vi "iIR.vi"(11 "PID gains":T1={"proportional gain (Kc)"=1.0, "integral time (Ti, min)"=0.01, "derivative time (Td, min)"=0.0} {"derivative time (Td, min)" format="%.4f"; "integral time (Ti, min)" format="%.3f"; "proportional gain (Kc)" format="%.3f"}) -> (2 "IR value":dbl[](array[numeric]), 9 "誤差":dbl)   [LabVIEW 2018]
uses:
  <vilib>/Platform/TimedLoop/XDataNode/timing_clust.ctl
  <vilib>/Platform/TimedLoop/XDataNode/nitl_modes.ctl
  <vilib>/Platform/TimedLoop/XDataNode/wakeup.ctl
  <vilib>/myRIO/Common/Instrument Driver Framework/myRIO v1.0/UART/vis/myRIO v1.0 Close UART.vi
  <vilib>/addons/control/pid/pid.llb/PID (DBL).vi
  <vilib>/myRIO/Common/Instrument Driver Framework/Utilities/vis/FPGA Ref Manager.vi
  <vilib>/myRIO/Common/Instrument Driver Framework/myRIO v1.0/myRIO v1.0 Reset FPGA.vi
  <vilib>/myRIO/Common/Instrument Driver Framework/myRIO v1.0/IRQ/vis/myRIO v1.0 IRQ Info FGV.vi
  <vilib>/myRIO/Common/Instrument Driver Framework/myRIO v1.0/IRQ/vis/myRIO v1.0 Timer IRQ Info FGV.vi
  <vilib>/myRIO/Common/Instrument Driver Framework/myRIO v1.0/IRQ/vis/myRIO v1.0 ISR Agent.vi
  <vilib>/platform/TimedLoop/XDataNode/XDataNode.xnode
  <vilib>/addons/control/pid/NI_PID_pid.lvlib
  <vilib>/Platform/TimedLoop/XDataNode/XDNodeRunTimeDep.lvlib
  <vilib>/myRIO/Instrument Drivers/Utilities/Utilities.lvlib
panel:
  in  "stop":bool
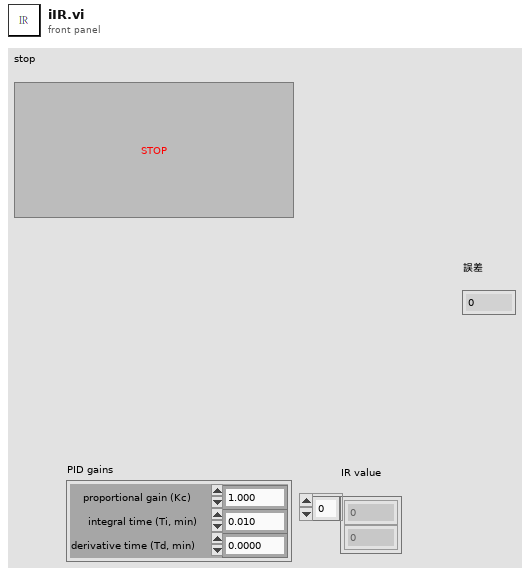
[diagram p1: front panel]
types:
  T1 = cluster{"proportional gain (Kc)":dbl, "integral time (Ti, min)":dbl, "derivative time (Td, min)":dbl}
  T2 = typedef "XDNodeRunTimeDep.lvlib/timing_clust.ctl" = cluster{"Expected End [f-1]":u64, "Actual End [f-1]":u64, "Finished Late? [f-1]":bool, "Expected End [i-1]":u64, "Actual End [i-1]":u64, "Finished Late? [i-1]":bool, "Expected Start [i]":u64, "Actual Start [i]":u64, "Expected Start [f]":u64, "Actual Start [f]":u64, "Source Name":string, "Structure Name":string, "Period":i64, "Deadline":i64, "Offset":i64, "Start":i64, "Priority":i32, "Timeout":i32, "Mode":T3, "Wakeup Reason":T4, "Error":errorcluster, "Source Type":string, "Secondary Source Type":string, "Global End Time":u64, "Global Start Time":u64, "Frame Duration":u64, "Iteration Duration":u64, "Assigned CPU":i32, "I/O Scan Engine Mode":u32}
  T3 = typedef "XDNodeRunTimeDep.lvlib/nitl_modes.ctl" = enum32{"No Change", "Process missed periods, maintain original phase", "Discard missed periods, maintain original phase", "Process missed periods, ignore original phase", "Discard missed periods, ignore original phase"}
  T4 = typedef "XDNodeRunTimeDep.lvlib/wakeup.ctl" = enum32{"Normal", "Aborted", "Asynchronous wakeup", "Timing source error", "Timed loop error", "Timeout"}
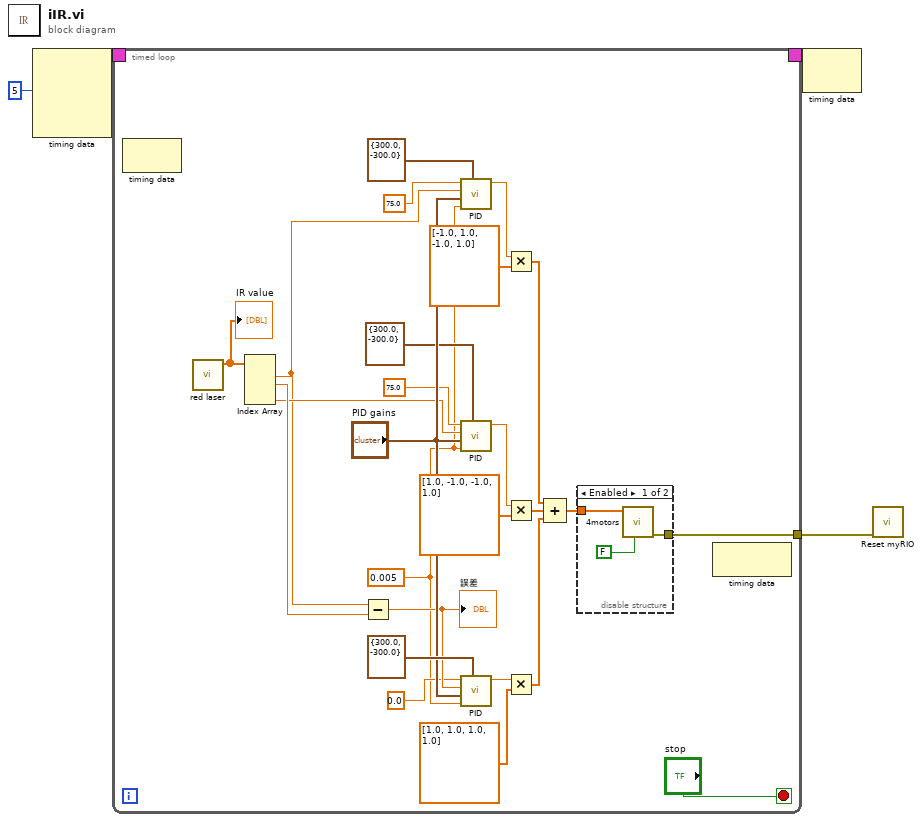
[diagram p0: block diagram]
diagram:
  n1 = node-c288(5) -> (w4:T2)  [unwired: 3 in]
  n2 = timed-loop {
    timing: w4 -> [_]
    timing-out: [_] -> w3
    tunnel: [w26] -> w1
    stop <- "stop" stop-if-true
    w5 = 0.005 ("dt (s)")
    n3 = node-c288() -> ()  [unwired: 1 in, 1 out]
    n4 = call "red laser.vi"() -> ("IR"=w29:dbl[])  [unwired: 10 in, 1 out]
    "IR value" <- w29
    n5 = Index Array(array=w29) -> (element #1=w6:dbl, element #2=w20:dbl, element #4=w13:dbl)  [unwired: 4 in, 1 out]
    n6 = Subtract(x=w6, y=w20) -> (x-y=w9:dbl)
    "誤差" <- w9
    n7 = call-poly <vilib>:"PID.vi"("output range"=cluster{"output high":dbl, "output low":dbl} {"output high"=300.0, "output low"=-300.0}, "dt (s)"=w5, "PID gains"="PID gains", "process variable"=w6, "setpoint"=75.0) -> ("output"=w22:dbl)  [unwired: 5 in, 1 out]
    n8 = call-poly <vilib>:"PID.vi"("output range"=cluster{"output high":dbl, "output low":dbl} {"output high"=300.0, "output low"=-300.0}, "dt (s)"=w5, "PID gains"="PID gains", "process variable"=w13, "setpoint"=75.0) -> ("output"=w14:dbl)  [unwired: 5 in, 1 out]
    n9 = call-poly <vilib>:"PID.vi"("output range"=cluster{"output high":dbl, "output low":dbl} {"output high"=300.0, "output low"=-300.0}, "dt (s)"=w5, "PID gains"="PID gains", "process variable"=w9, "setpoint"=0.0) -> ("output"=w23:dbl)  [unwired: 5 in, 1 out]
    n10 = Multiply(x=w22, y=dbl[] [-1.0, 1.0, -1.0, 1.0]) -> (x*y=w11:dbl[])
    n11 = Multiply(x=w14, y=dbl[] [1.0, -1.0, -1.0, 1.0]) -> (x*y=w12:dbl[])
    n12 = Multiply(x=w23, y=dbl[] [1.0, 1.0, 1.0, 1.0]) -> (x*y=w7:dbl[])
    n13 = Compound Arithmetic op=ADD(w11, w12, w7) -> (w10:dbl[])
    n14 = disable-structure shown="Enabled" {
      disable-tunnel: [w32 _] -> w26
      disable-tunnel: w10 -> [w30 _]
      frame Enabled {
        n15 = call "4motors.vi"("Reset"=FALSE, "Power"=w30) -> ("error out"=w32:errorcluster)  [unwired: 8 in, 1 out]
      }
      frame Disabled {
      }
    }
    n16 = node-c288() -> ()  [unwired: 1 in, 1 out]
  }
  n17 = node-c288(w3) -> ()  [unwired: 1 out]
  n18 = call <vilib>:"Reset myRIO.vi"("error in (no error)"=w1) -> ()  [unwired: 10 in, 1 out]
